vi "CenterRobot.vi"(9 "manual control":dbl, 10 "process variable":dbl, 11 "setpoint":dbl) -> (3 "output":dbl)   [LabVIEW 2016]
uses:
  <vilib>/addons/control/pid/autopid.llb/PID autotuning parameters (adv).ctl
  <vilib>/addons/control/pid/pid.llb/PID Lead-Lag (DBL).vi
  <vilib>/addons/control/pid/NI_PID_autopid.lvlib
  <vilib>/addons/control/pid/NI_PID_pid.lvlib
panel:
  in  "output range":cluster{"output high":dbl, "output low":dbl}={"output high"=0.7, "output low"=-0.7}
  in  "tuning parameters":T1={"gain"=1.0, "lag time"=0.5, "lead time"=0.0}
  in  "gamma":dbl format="%.2f"
  out "tuned PID gains":T2={"proportional gain (Kc)"=1.0, "integral time (Ti, min)"=0.01, "derivative time (Td, min)"=0.0} {"derivative time (Td, min)" format="%#.6g"; "integral time (Ti, min)" format="%#.6g"; "proportional gain (Kc)" format="%#.6g"}
  out "tuning completed?":bool
  in  "autotuning parameters":T3={"technique"=2, "type of controller"=1, "control specification"=0, "amplitude"=1.0} {"amplitude" format="%.2f"; "control specification" items=["normal", "fast", "slow"]; "type of controller" items=["P", "PI", "PID"]; "technique" items=["Step Open Loop", "Step Closed Loop", "Relay", "PID Relay"]}
  in  "PID gains":T2={"proportional gain (Kc)"=0.8, "integral time (Ti, min)"=0.01, "derivative time (Td, min)"=0.0} {"derivative time (Td, min)" format="%#.6g"; "integral time (Ti, min)" format="%#.6g"; "proportional gain (Kc)" format="%#.6g"}
  in  "autotune? (F)":bool
  in  "auto? (F)":bool=TRUE
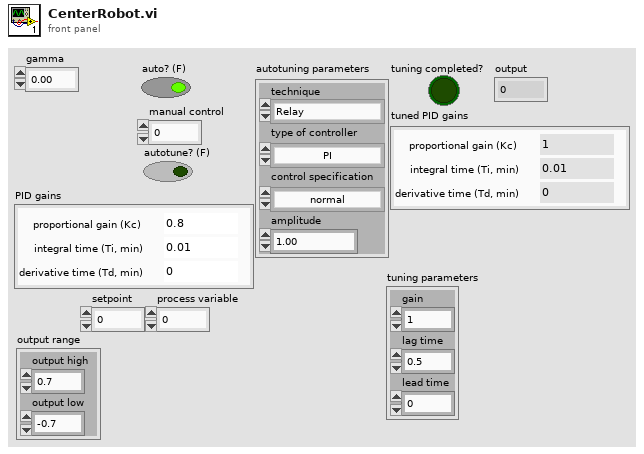
[diagram p1: front panel]
types:
  T1 = cluster{"gain":dbl, "lag time":dbl, "lead time":dbl}
  T2 = cluster{"proportional gain (Kc)":dbl, "integral time (Ti, min)":dbl, "derivative time (Td, min)":dbl}
  T3 = typedef "NI_PID_autopid.lvlib/PID autotuning parameters (adv).ctl" = cluster{"technique":u16, "type of controller":u16, "control specification":u16, "amplitude":dbl}
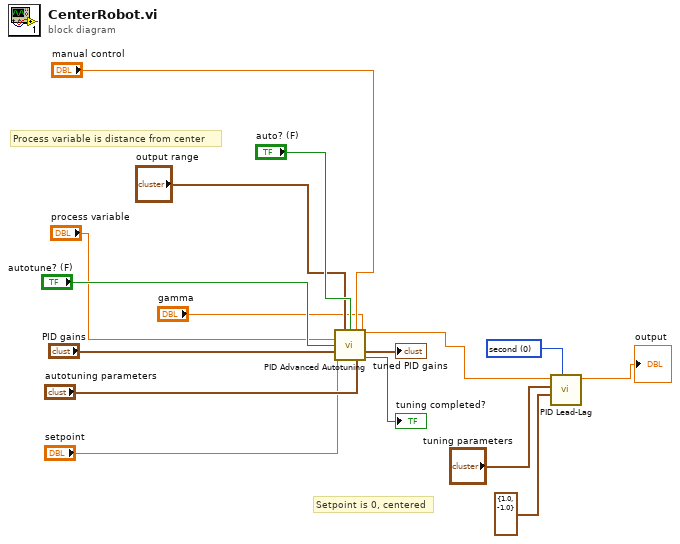
[diagram p0: block diagram]
diagram:
  w5 = u16 0 items=["second", "minute"] ("time unit")
  # "Setpoint is 0, centered"
  # "Process variable is distance from center"
  n1 = call <vilib>:"PID Advanced Autotuning.vi"("setpoint"="setpoint", "output range"="output range", "auto? (F)"="auto? (F)", "manual control"="manual control", "process variable"="process variable", "gamma"="gamma", "autotune? (F)"="autotune? (F)", "PID gains"="PID gains", "autotuning parameters"="autotuning parameters") -> ("output"=w3:dbl, "tuned PID gains"=→"tuned PID gains":T2, "tuning completed?"=→"tuning completed?":bool)  [unwired: 4 in]
  n2 = call-poly <vilib>:"PID Lead-Lag.vi"("time unit"=w5, "output range"=cluster{"output high":dbl, "output low":dbl} {"output high"=1.0, "output low"=-1.0}, "tuning parameters"="tuning parameters", "input"=w3) -> ("output"=→"output":dbl)  [unwired: 4 in, 1 out]
